vi "check tour is continuous.vi"(1 "tour":T1[](array[typedef])) -> (0 "T = the tour is continuous":bool)   [LabVIEW 2018, in "main.lvlib"]
uses:
  main.lvlib
  core/core_data/chessboard_index.ctl
  core/core.lvlib
  core/core_data/core_data.lvlib
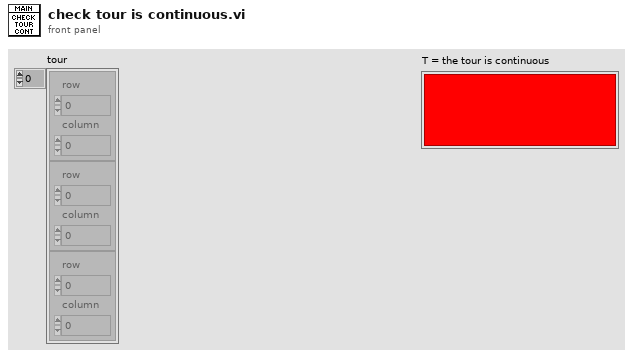
[diagram p1: front panel]
types:
  T1 = typedef "core.lvlib/core_data.lvlib/chessboard_index.ctl" = cluster{"row":u8, "column":u8}
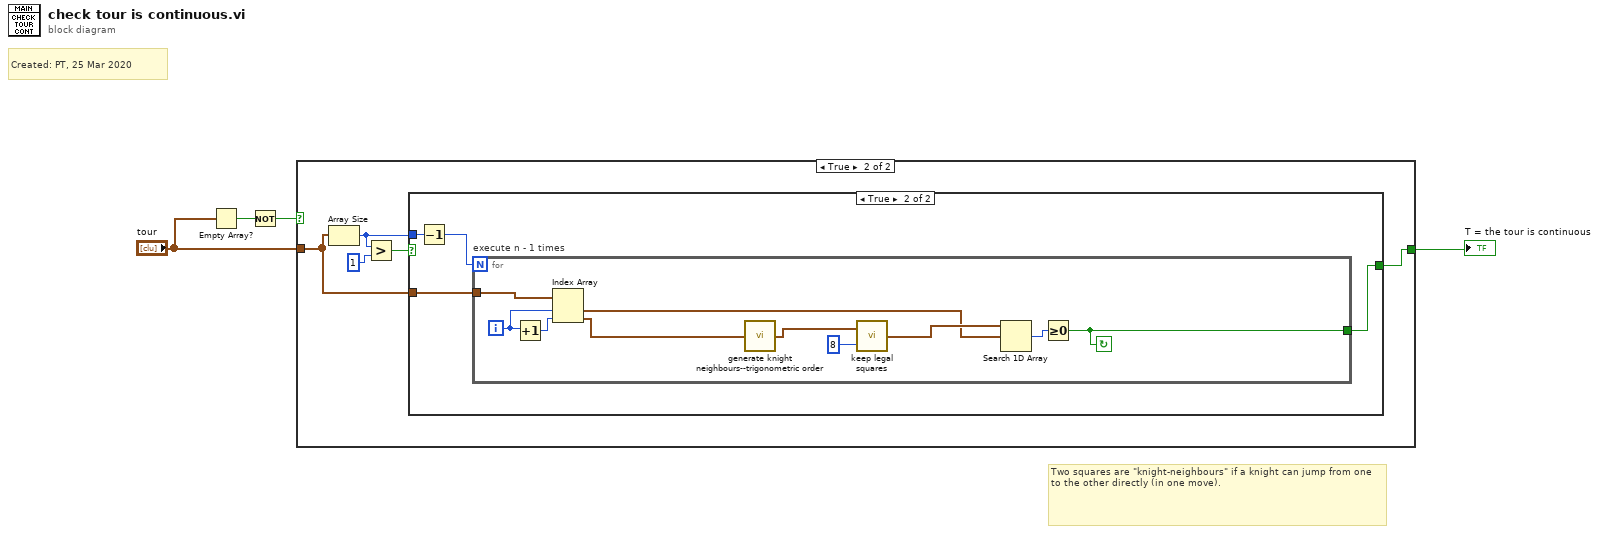
[diagram p0: block diagram]
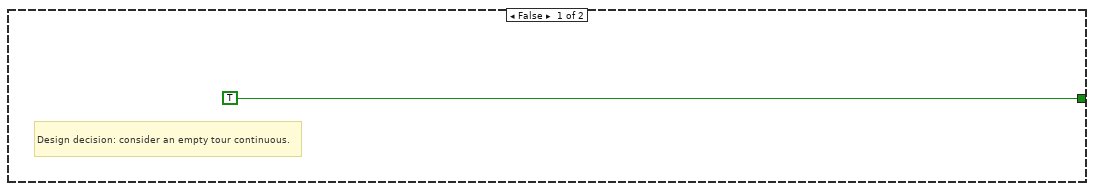
[diagram p2: hidden frame]
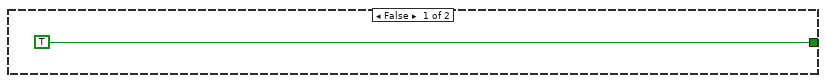
[diagram p3: hidden frame]
diagram:
  # "Two squares are \"knight-neighbours\" if a knight can jump from one to the other directly (in one move)."
  # "Created: PT, 25 Mar 2020"
  n1 = Empty Array?(array="tour") -> (empty?=w4:bool)
  n2 = Not(x=w4) -> (.not. x?=w3:bool)
  n3 = case shown="True" w3 {
    tunnel: [TRUE w8] -> w2
    tunnel: "tour" -> [_ w7]
    frame False {
      # "Design decision: consider an empty tour continuous."
    }
    frame True {
      n4 = Array Size(array=w7) -> (size(s)=w6:i32)
      n5 = Greater?(x=w6, y=1) -> (0:w10:bool)
      n6 = case shown="True" w10 {
        tunnel: [TRUE w12] -> w8
        tunnel: w7 -> [_ w15]
        tunnel: w6 -> [_ w14]
        frame False {
        }
        frame True {
          n7 = Decrement(x=w14) -> (x-1=w13:i32)
          n8 = for "execute n - 1 times" {
            N: w13 -> [_]
            tunnel: w15 -> [w25]
            tunnel: [w16] -> w12
            i -> [w24]
            stop <- w16 continue-if-true
            n9 = Increment(x=w24) -> (x+1=w23:i32)
            n10 = Index Array(array=w25, index #1=w24, index #2=w23) -> (element #1=w18:T1, element #2=w21:T1)
            n11 = call "generate knight neighbours--trigonometric order.vi"("current square (chessboard_index)"=w21) -> ("neighbours (chessboard_index)"=w22:T1[])
            n12 = call "keep legal squares.vi"("chessboard_size"=u8 8, "squares (chessboard_index)"=w22) -> ("legal squares only (chessboard_index)"=w19:T1[])
            n13 = Search 1D Array(1D array=w19, element=w18) -> (index of element=w17:i32)  [unwired: 1 in]
            n14 = Greater Or Equal To 0?(x=w17) -> (x >= 0?=w16:bool)
          }
        }
      }
    }
  }
  "T = the tour is continuous" <- w2
